vi "siAll Func Reverse Order Signed Long Bytes (I32).vi"(1 "Input I32 to convert":i32) -> (0 "Output I32 with byte order reversed":i32)   [LabVIEW 2015, in "XYZStage.lvlib"]
uses:
  XYZStage.lvlib
panel:
  out "Byte count on input":u8
  out "Byte count on output":u8
  out "Output bytes in hex":string
  out "Input bytes in hex":string
  # "Sutter Instrument's general-purpose function to reverse the order of bytes within a unsigned long (32-bits)."
  # "INPUT"
  # "OUTPUT"
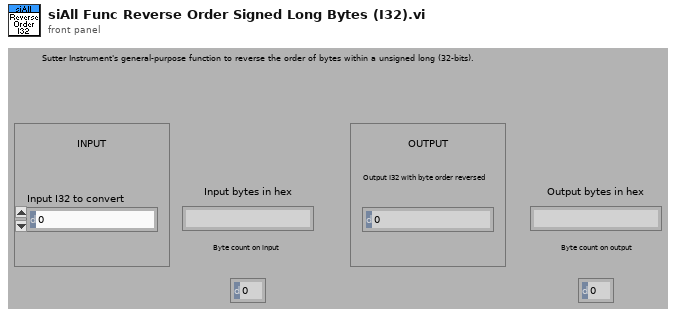
[diagram p1: front panel]
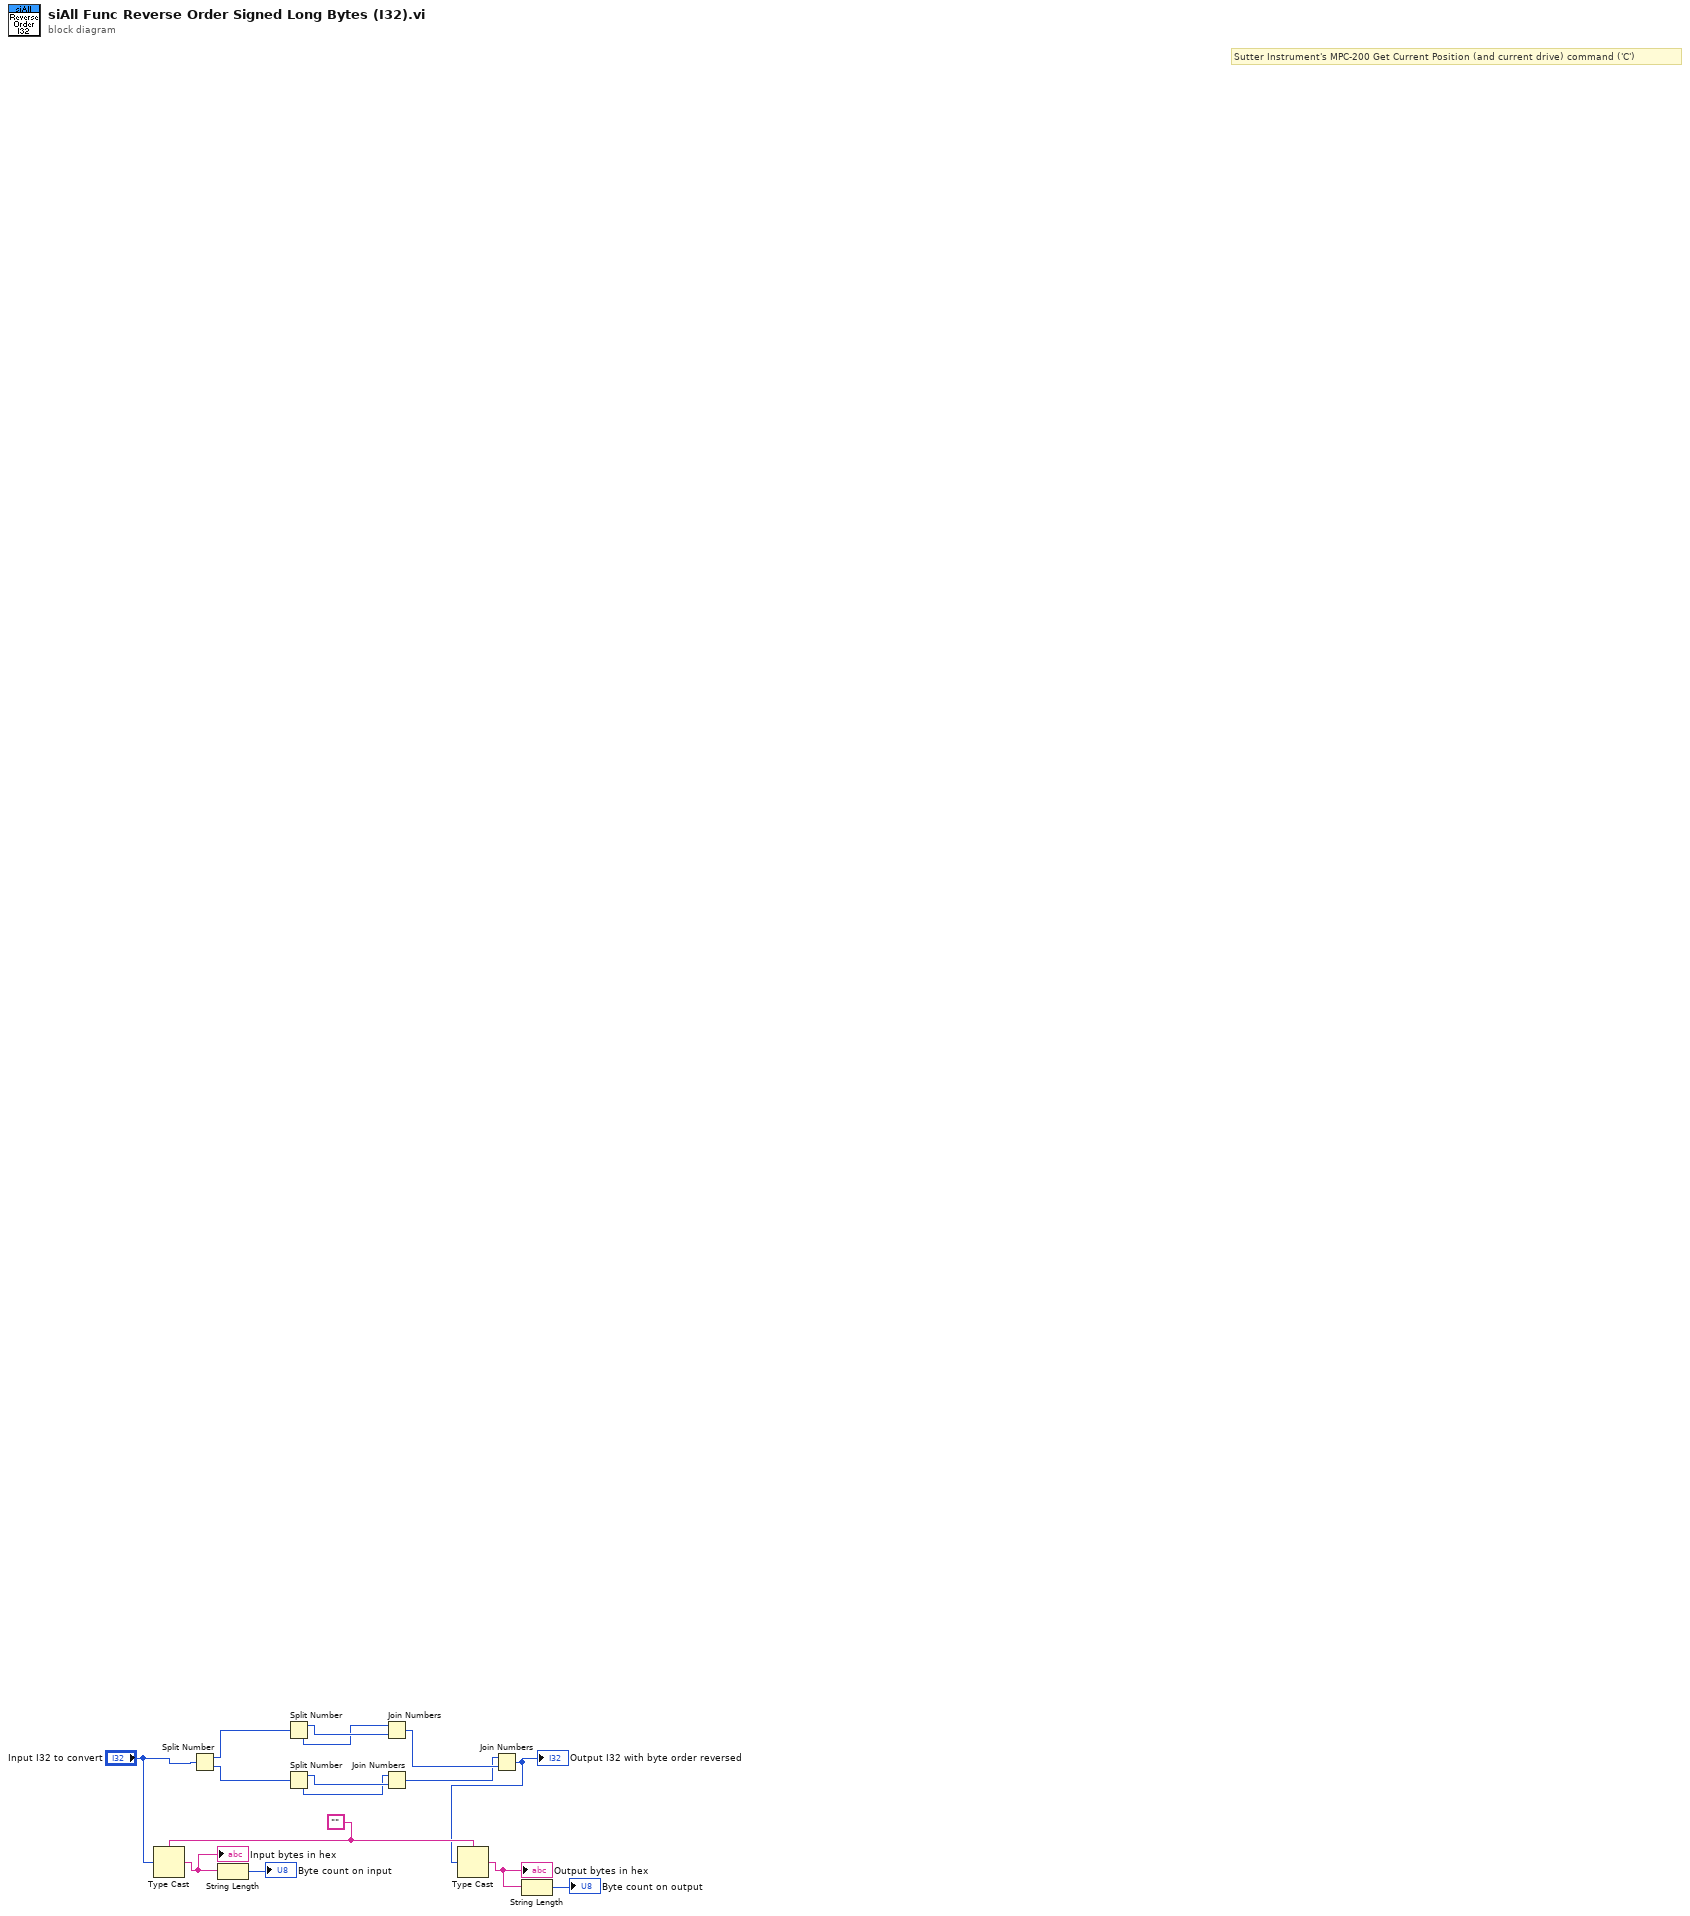
[diagram p0: block diagram]
diagram:
  w11 = ""
  # "Sutter Instrument's MPC-200 Get Current Position (and current drive) command ('C')"
  n1 = Type Cast(type=w11, x="Input I32 to convert") -> (*(type *) &x=w13:string)
  "Input bytes in hex" <- w13
  n2 = Split Number(x="Input I32 to convert") -> (hi(x)=w10:u16, lo(x)=w3:u16)
  n3 = String Length(string=w13) -> (length=→"Byte count on input":i32)
  n4 = Split Number(x=w10) -> (hi(x)=w9:u8, lo(x)=w8:u8)
  n5 = Split Number(x=w3) -> (hi(x)=w7:u8, lo(x)=w6:u8)
  n6 = Join Numbers(hi=w8, lo=w9) -> ((hi.lo)=w5:u16)
  n7 = Join Numbers(hi=w6, lo=w7) -> ((hi.lo)=w4:u16)
  n8 = Join Numbers(hi=w4, lo=w5) -> ((hi.lo)=w2:u32)
  "Output I32 with byte order reversed" <- w2
  n9 = Type Cast(type=w11, x=w2) -> (*(type *) &x=w14:string)
  "Output bytes in hex" <- w14
  n10 = String Length(string=w14) -> (length=→"Byte count on output":i32)
